vi "Variant Functional Globals.vi"(9 "State":enum16{"Get", "Set"}(ring), 10 "Data":variant) -> (2 "Data Out":variant)   [LabVIEW 2014]
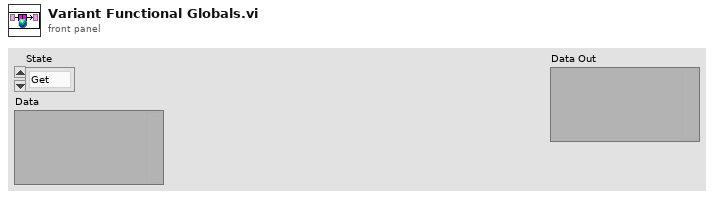
[diagram p1: front panel]
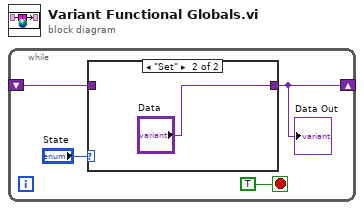
[diagram p0: block diagram]
diagram:
  n1 = while {
    shift-right: [w1] -> _
    shift-left: _ -> [w2]
    stop <- TRUE stop-if-true
    n2 = case shown="\"Set\"" "State" {
      tunnel: w2 -> [w5 _]
      tunnel: [w5 "Data"] -> w1
      frame "Get", Default {
      }
      frame "Set" {
      }
    }
    "Data Out" <- w1
  }
